vi "SubTRAMAS.vi"(0 "Trama":string) -> (1 "RMC":string[](array[string]), 2 "GGA":string[](array[string]), 3 "GSA":string[](array[string]))   [LabVIEW 2020]
panel:
  out "<CR><LF> GSA":string
  out "<CR><LF> GGA":string
  out "<CR><LF> RMC":string
  out "Estado de navegación RMC":string
  out "Longitud GGA":string
  out "Latitud GGA":string
  out "Longitud RMC":string
  out "Latitud RMC":string
  out "Dilución vertical de precisión GSA":string
  out "Checksum GSA":string
  out "Checksum GGA":string
  out "ID de la estación DGPS GGA":string
  out "Edad DGPS GGA":string
  out "Checksum RMC":string
  out "ID del sistema GNSS GSA":string
  out "Dilución horizontal de precisión GSA":string
  out "Posición dilución de precisión GSA":string
  out "Satelite usado en el canal 12":string
  out "Satelite usado en el canal 11":string
  out "Satelite usado en el canal 10":string
  out "Satelite usado en el canal 9":string
  out "Satelite usado en el canal 8":string
  out "Satelite usado en el canal 7":string
  out "Satelite usado en el canal 6":string
  out "Satelite usado en el canal 5":string
  out "Satelite usado en el canal 4":string
  out "Satelite usado en el canal 3":string
  out "Satelite usado en el canal 2":string
  out "Satelite usado en el canal 1":string
  out "Fix status GSA":string
  out "Modo":string
  out "Separacion geoide GGA":string
  out "Altitud GGA":string
  out "Fix Status GGA":string
  out "Modo de posicionamiento RMC":string
  out "Variacion magnetica RMC":string
  out "Variacion  RMC":string
  out "COG RMC":string
  out "HDOP GGA":string
  out "dds 2":dbl
  out "ma 2":dbl
  out "N° satelites en uso GGA":string
  out "Tiempo GGA":string
  out "dds":dbl
  out "ma":dbl
  out "Valida o Invalida? RMC":string
  out "Velocidad RMC":string
  out "Tiempo RMC":string
  out "Fecha RMC":string
  # "RMC"
  # "GGA"
  # "GSA"
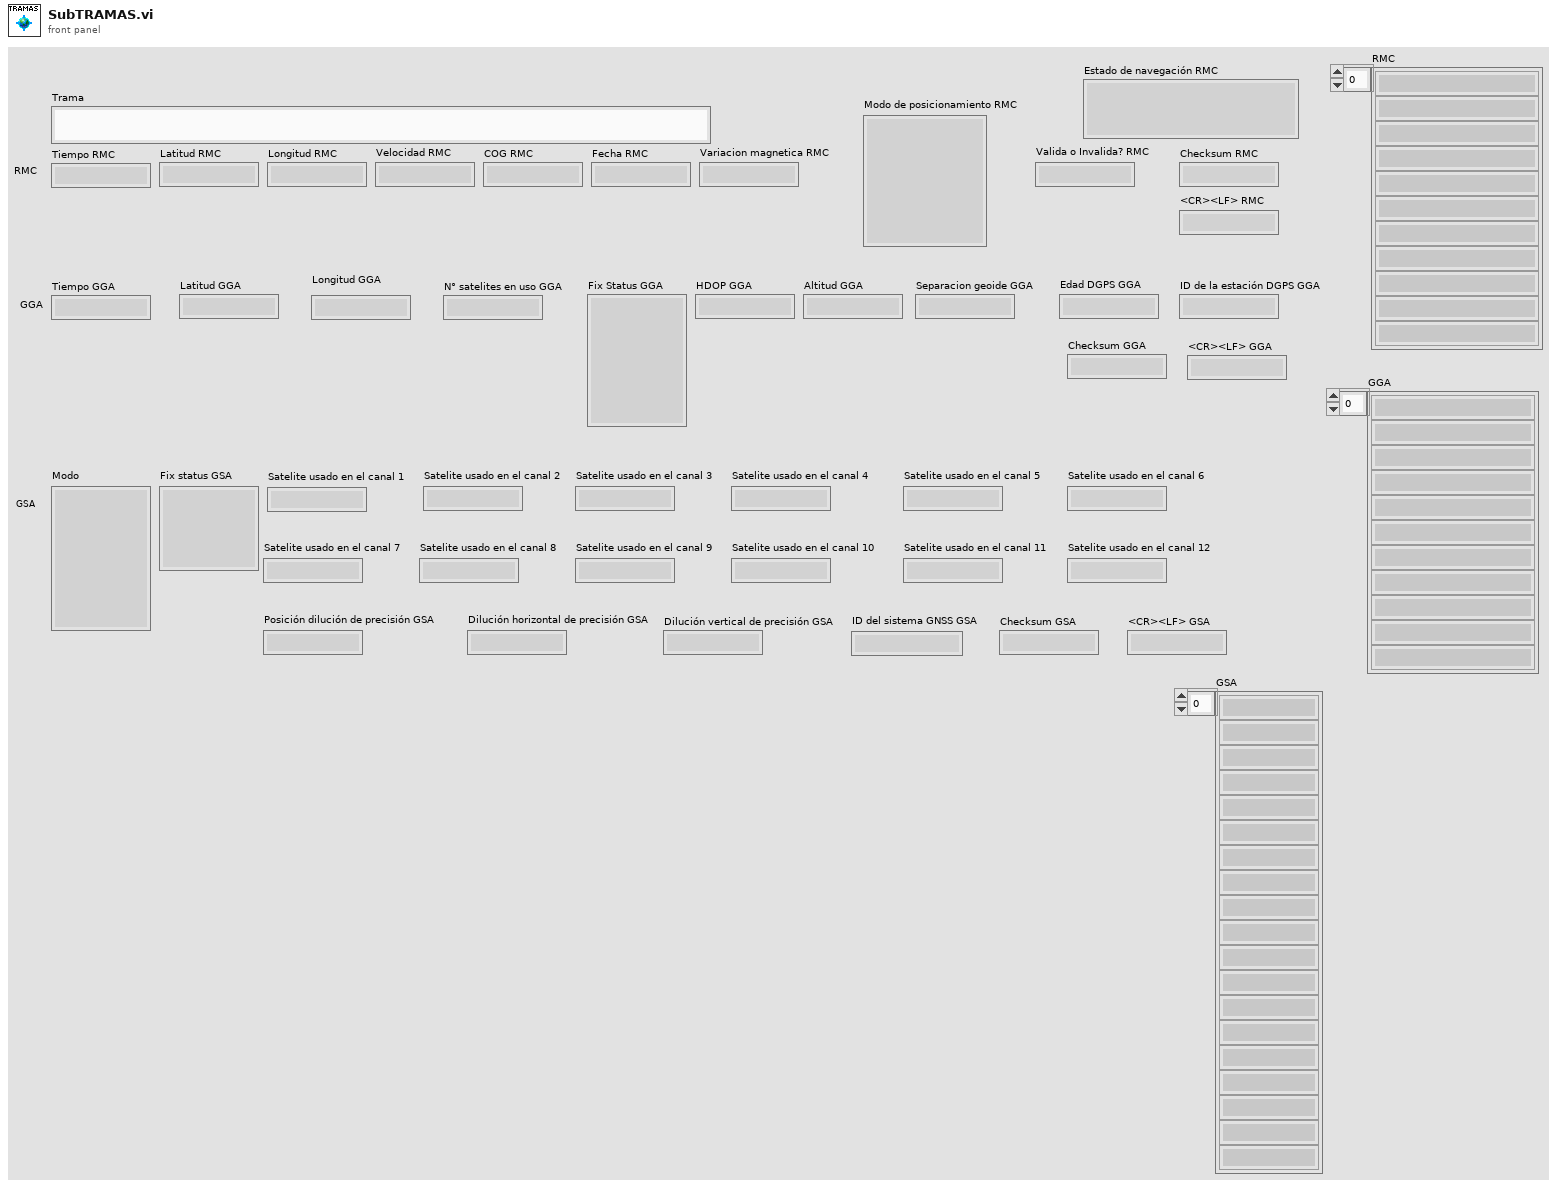
[diagram p1: front panel]
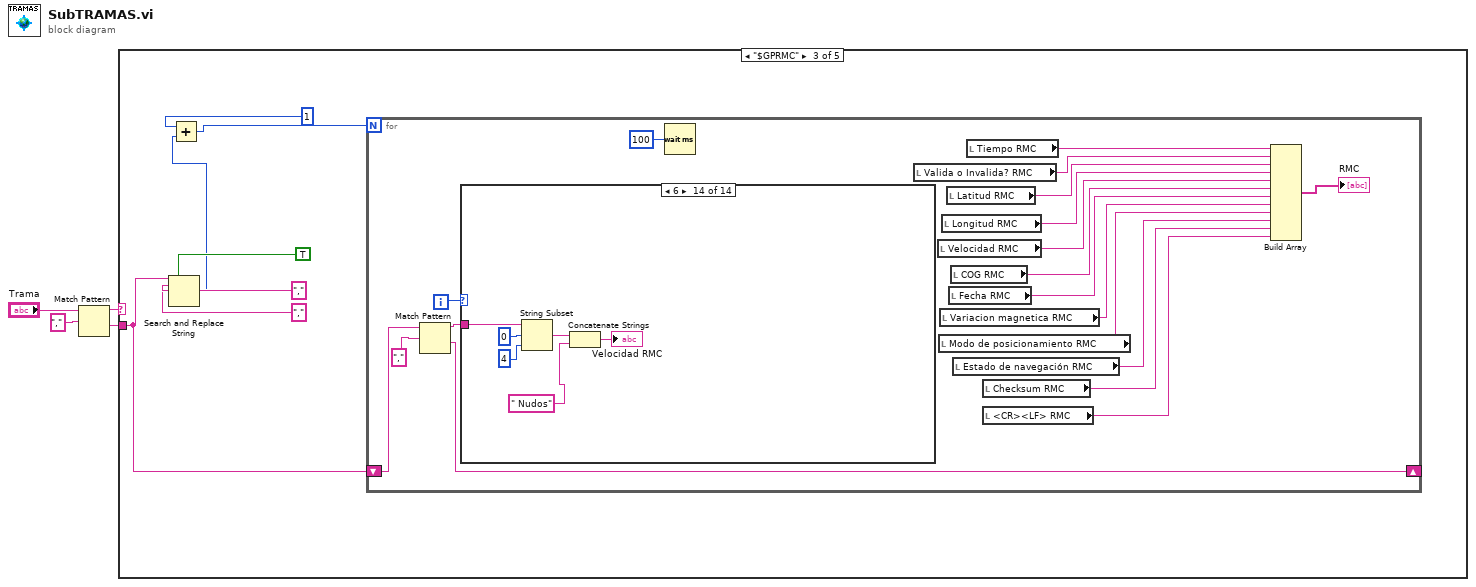
[diagram p0: block diagram]
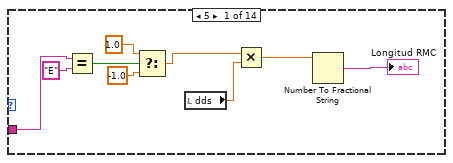
[diagram p4: hidden frame]
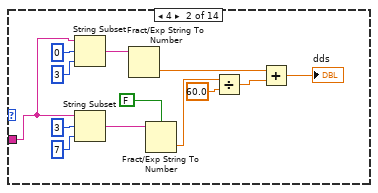
[diagram p5: hidden frame]
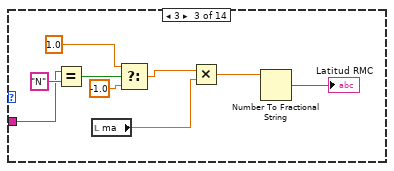
[diagram p6: hidden frame]
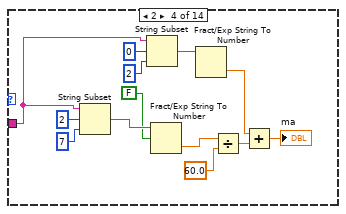
[diagram p7: hidden frame]
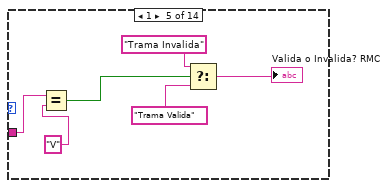
[diagram p8: hidden frame]
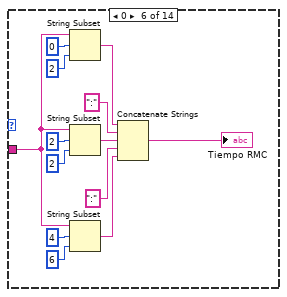
[diagram p9: hidden frame]
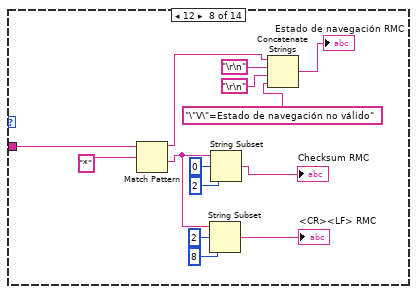
[diagram p11: hidden frame]
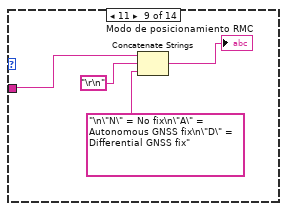
[diagram p12: hidden frame]
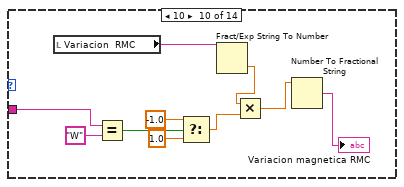
[diagram p13: hidden frame]
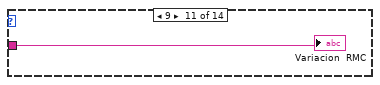
[diagram p14: hidden frame]
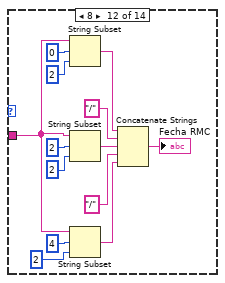
[diagram p15: hidden frame]
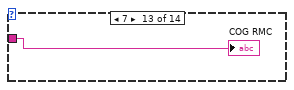
[diagram p16: hidden frame]
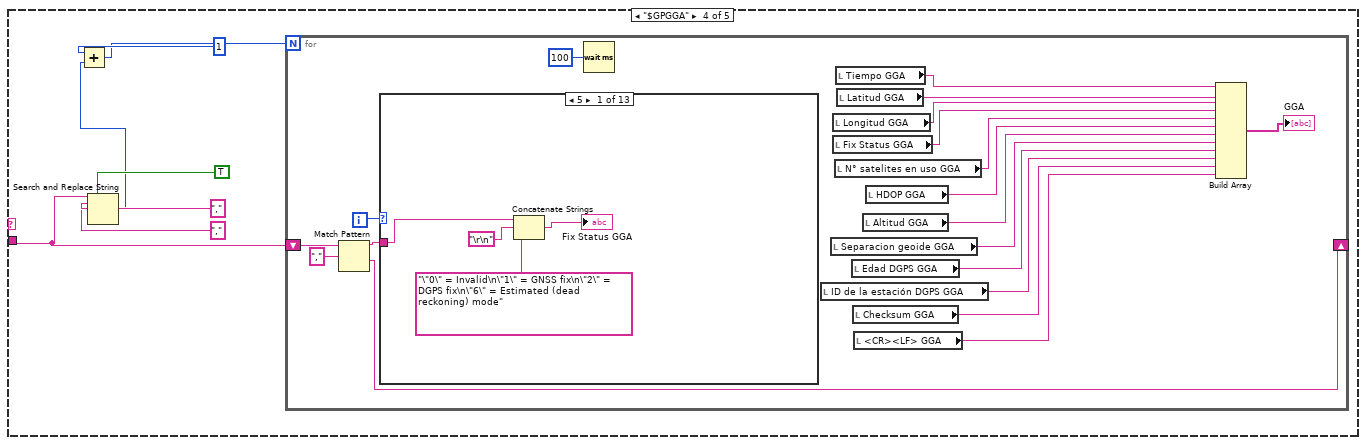
[diagram p17: hidden frame]
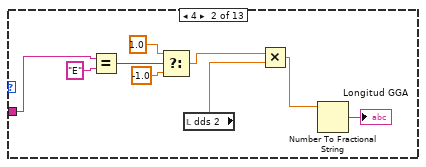
[diagram p18: hidden frame]
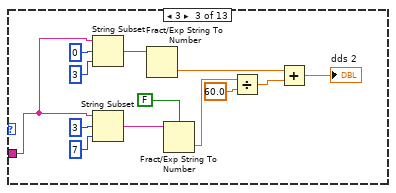
[diagram p19: hidden frame]
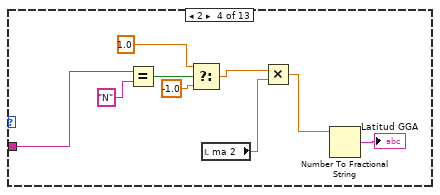
[diagram p20: hidden frame]
diagram:
  n1 = Match Pattern(string="Trama", regular expression=",") -> (before substring=w3:string, after substring=w2:string)  [unwired: 1 in, 2 out]
  n2 = case shown="\"$GPRMC\"" w3 {
    tunnel: w2 -> [_ _ w9 w146 w248]
    frame "False", Default {
    }
    frame "True" {
    }
    frame "$GPRMC" {
      n3 = Search and Replace String(replace all?=TRUE ("replace all? (F)"), input string=w9, search string=",", replace string="," ("replace string (\"\")")) -> (number of replacements=w6:i32)  [unwired: 4 in, 3 out]
      n4 = Add(x=1, y=w6) -> (x+y=w5:i32)
      n5 = for {
        N: w5 -> [_]
        shift-right: [w26] -> _
        shift-left: w9 -> [w29]
        i -> [w28]
        n6 = Match Pattern(string=w29, regular expression=",") -> (before substring=w27:string, after substring=w26:string)  [unwired: 1 in, 2 out]
        n7 = case shown="6" w28 {
          tunnel: w27 -> [w34 w41 w58 w63 w77 w82 _ w106 w110 w116 w122 w124 w136 w138]
          frame 5 {
            n8 = Equal?(x=w34, y="E") -> (x = y?=w37:bool)
            n9 = Select(t=1.0, s=w37, f=-1.0) -> (s? t:f=w35:dbl)
            n10 = local read "dds"() -> (w33:dbl)
            n11 = Multiply(x=w35, y=w33) -> (x*y=w32:dbl)
            n12 = Number To Fractional String(number=w32) -> (F-format string=→"Longitud RMC":string)  [unwired: 3 in]
          }
          frame 4 {
            n13 = String Subset(string=w41, offset (0)=0, length (rest)=3 ("length (rest)")) -> (substring=w52:string)
            n14 = String Subset(string=w41, offset (0)=3, length (rest)=7 ("length (rest)")) -> (substring=w48:string)
            n15 = Fract/Exp String To Number(string=w52) -> (number=w43:dbl)  [unwired: 3 in, 1 out]
            n16 = Fract/Exp String To Number(use system decimal point (T)=FALSE, string=w48) -> (number=w50:dbl)  [unwired: 2 in, 1 out]
            n17 = Divide(x=w50, y=60.0) -> (x/y=w42:dbl)
            n18 = Add(x=w43, y=w42) -> (x+y=→"dds":dbl)
          }
          frame 3 {
            n19 = Equal?(x=w58, y="N") -> (x = y?=w60:bool)
            n20 = local read "ma"() -> (w55:dbl)
            n21 = Select(t=1.0, s=w60, f=-1.0) -> (s? t:f=w56:dbl)
            n22 = Multiply(x=w56, y=w55) -> (x*y=w54:dbl)
            n23 = Number To Fractional String(number=w54) -> (F-format string=→"Latitud RMC":string)  [unwired: 3 in]
          }
          frame 2 {
            n24 = String Subset(string=w63, offset (0)=2, length (rest)=7 ("length (rest)")) -> (substring=w70:string)
            n25 = String Subset(string=w63, offset (0)=0, length (rest)=2 ("length (rest)")) -> (substring=w65:string)
            n26 = Fract/Exp String To Number(use system decimal point (T)=FALSE, string=w70) -> (number=w68:dbl)  [unwired: 2 in, 1 out]
            n27 = Fract/Exp String To Number(string=w65) -> (number=w64:dbl)  [unwired: 3 in, 1 out]
            n28 = Divide(x=w68, y=60.0) -> (x/y=w66:dbl)
            n29 = Add(x=w64, y=w66) -> (x+y=→"ma":dbl)
          }
          frame 1 {
            n30 = Equal?(x=w77, y="V") -> (x = y?=w75:bool)
            n31 = Select(t="Trama Invalida", s=w75, f="Trama Valida") -> (s? t:f=→"Valida o Invalida? RMC":string)
          }
          frame 0 {
            n32 = String Subset(string=w82, offset (0)=0, length (rest)=2 ("length (rest)")) -> (substring=w87:string)
            n33 = String Subset(string=w82, offset (0)=2, length (rest)=2 ("length (rest)")) -> (substring=w85:string)
            n34 = String Subset(string=w82, offset (0)=4, length (rest)=6 ("length (rest)")) -> (substring=w83:string)
            n35 = Concatenate Strings(w87, ":" ("string"), w85, ":" ("string"), w83) -> (→"Tiempo RMC":string)
          }
          frame 20, Default {
          }
          frame 12 {
            n36 = Match Pattern(string=w106, regular expression="*") -> (before substring=w102:string, after substring=w100:string)  [unwired: 1 in, 2 out]
            n37 = String Subset(string=w100, offset (0)=2, length (rest)=8 ("length (rest)")) -> (substring=→"<CR><LF> RMC":string)
            n38 = String Subset(string=w100, offset (0)=0, length (rest)=2 ("length (rest)")) -> (substring=→"Checksum RMC":string)
            n39 = Concatenate Strings(w102, "\r\n", "\r\n", "\"V\"=Estado de navegación no válido") -> (→"Estado de navegación RMC":string)
          }
          frame 11 {
            n40 = Concatenate Strings(w110, "\r\n", "\n\"N\" = No fix\n\"A\" = Autonomous GNSS fix\n\"D\" = Differential GNSS fix") -> (→"Modo de posicionamiento RMC":string)
          }
          frame 10 {
            n41 = local read "Variacion  RMC"() -> (w115:string)
            n42 = Equal?(x=w116, y="W") -> (x = y?=w120:bool)
            n43 = Select(t=-1.0, s=w120, f=1.0) -> (s? t:f=w117:dbl)
            n44 = Fract/Exp String To Number(string=w115) -> (number=w114:dbl)  [unwired: 3 in, 1 out]
            n45 = Multiply(x=w114, y=w117) -> (x*y=w113:dbl)
            n46 = Number To Fractional String(number=w113) -> (F-format string=→"Variacion magnetica RMC":string)  [unwired: 3 in]
          }
          frame 9 {
            "Variacion  RMC" <- w122
          }
          frame 8 {
            n47 = String Subset(string=w124, offset (0)=0, length (rest)=2 ("length (rest)")) -> (substring=w130:string)
            n48 = String Subset(string=w124, offset (0)=2, length (rest)=2 ("length (rest)")) -> (substring=w128:string)
            n49 = String Subset(string=w124, offset (0)=4, length (rest)=2 ("length (rest)")) -> (substring=w126:string)
            n50 = Concatenate Strings(w130, "/" ("string"), w128, "/" ("string"), w126) -> (→"Fecha RMC":string)
          }
          frame 7 {
            "COG RMC" <- w136
          }
          frame 6 {
            n51 = String Subset(string=w138, offset (0)=0, length (rest)=4 ("length (rest)")) -> (substring=w140:string)
            n52 = Concatenate Strings(w140, " Nudos") -> (→"Velocidad RMC":string)
          }
        }
        n53 = Wait (ms)(milliseconds to wait=u32 100) -> ()  [unwired: 1 out]
        n54 = local read "Valida o Invalida? RMC"() -> (w22:string)
        n55 = local read "Velocidad RMC"() -> (w19:string)
        n56 = local read "Modo de posicionamiento RMC"() -> (w15:string)
        n57 = local read "Variacion magnetica RMC"() -> (w16:string)
        n58 = local read "Longitud RMC"() -> (w20:string)
        n59 = local read "Latitud RMC"() -> (w21:string)
        n60 = local read "Fecha RMC"() -> (w17:string)
        n61 = local read "COG RMC"() -> (w18:string)
        n62 = local read "Estado de navegación RMC"() -> (w14:string)
        n63 = local read "Tiempo RMC"() -> (w24:string)
        n64 = local read "Checksum RMC"() -> (w13:string)
        n65 = local read "<CR><LF> RMC"() -> (w12:string)
        n66 = Build Array(w24, w22, w21, w20, w19, w18, w17, w16, w15, w14, w13, w12) -> (→"RMC":string[])
      }
    }
    frame "$GPGGA" {
      n67 = Search and Replace String(replace all?=TRUE ("replace all? (F)"), input string=w146, search string=",", replace string="," ("replace string (\"\")")) -> (number of replacements=w144:i32)  [unwired: 4 in, 3 out]
      n68 = Add(x=1, y=w144) -> (x+y=w143:i32)
      n69 = for {
        N: w143 -> [_]
        shift-right: [w164] -> _
        shift-left: w146 -> [w167]
        i -> [w166]
        n70 = Match Pattern(string=w167, regular expression=",") -> (before substring=w165:string, after substring=w164:string)  [unwired: 1 in, 2 out]
        n71 = case shown="5" w166 {
          tunnel: w165 -> [w172 w176 w182 w198 w209 w217 _ w238 w240 w241 w242 w243 w244]
          frame 5 {
            n72 = Concatenate Strings(w172, "\r\n", "\"0\" = Invalid\n\"1\" = GNSS fix\n\"2\" = DGPS fix\n\"6\" = Estimated (dead reckoning) mode") -> (→"Fix Status GGA":string)
          }
          frame 4 {
            n73 = Equal?(x=w176, y="E") -> (x = y?=w179:bool)
            n74 = Select(t=1.0, s=w179, f=-1.0) -> (s? t:f=w177:dbl)
            n75 = local read "dds 2"() -> (w175:dbl)
            n76 = Multiply(x=w177, y=w175) -> (x*y=w174:dbl)
            n77 = Number To Fractional String(number=w174) -> (F-format string=→"Longitud GGA":string)  [unwired: 3 in]
          }
          frame 3 {
            n78 = String Subset(string=w182, offset (0)=0, length (rest)=3 ("length (rest)")) -> (substring=w194:string)
            n79 = String Subset(string=w182, offset (0)=3, length (rest)=7 ("length (rest)")) -> (substring=w190:string)
            n80 = Fract/Exp String To Number(string=w194) -> (number=w185:dbl)  [unwired: 3 in, 1 out]
            n81 = Fract/Exp String To Number(use system decimal point (T)=FALSE, string=w190) -> (number=w192:dbl)  [unwired: 2 in, 1 out]
            n82 = Divide(x=w192, y=60.0) -> (x/y=w184:dbl)
            n83 = Add(x=w185, y=w184) -> (x+y=→"dds 2":dbl)
          }
          frame 2 {
            n84 = Equal?(x=w198, y="N") -> (x = y?=w202:bool)
            n85 = Select(t=1.0, s=w202, f=-1.0) -> (s? t:f=w199:dbl)
            n86 = local read "ma 2"() -> (w197:dbl)
            n87 = Multiply(x=w199, y=w197) -> (x*y=w196:dbl)
            n88 = Number To Fractional String(number=w196) -> (F-format string=→"Latitud GGA":string)  [unwired: 3 in]
          }
          frame 1 {
            n89 = String Subset(string=w209, offset (0)=2, length (rest)=7 ("length (rest)")) -> (substring=w214:string)
            n90 = String Subset(string=w209, offset (0)=0, length (rest)=2 ("length (rest)")) -> (substring=w211:string)
            n91 = Fract/Exp String To Number(use system decimal point (T)=FALSE, string=w214) -> (number=w213:dbl)  [unwired: 2 in, 1 out]
            n92 = Fract/Exp String To Number(string=w211) -> (number=w208:dbl)  [unwired: 3 in, 1 out]
            n93 = Divide(x=w213, y=60.0) -> (x/y=w212:dbl)
            n94 = Add(x=w208, y=w212) -> (x+y=→"ma 2":dbl)
          }
          frame 0 {
            n95 = String Subset(string=w217, offset (0)=0, length (rest)=2 ("length (rest)")) -> (substring=w223:string)
            n96 = String Subset(string=w217, offset (0)=2, length (rest)=2 ("length (rest)")) -> (substring=w221:string)
            n97 = String Subset(string=w217, offset (0)=4, length (rest)=6 ("length (rest)")) -> (substring=w219:string)
            n98 = Concatenate Strings(w223, ":" ("string"), w221, ":" ("string"), w219) -> (→"Tiempo GGA":string)
          }
          frame 15, Default {
          }
          frame 13 {
            n99 = Match Pattern(string=w238, regular expression="*") -> (before substring=→"ID de la estación DGPS GGA":string, after substring=w230:string)  [unwired: 1 in, 2 out]
            n100 = String Subset(string=w230, offset (0)=2, length (rest)=8 ("length (rest)")) -> (substring=→"<CR><LF> GGA":string)
            n101 = String Subset(string=w230, offset (0)=0, length (rest)=2 ("length (rest)")) -> (substring=→"Checksum GGA":string)
          }
          frame 12 {
            "Edad DGPS GGA" <- w240
          }
          frame 10 {
            "Separacion geoide GGA" <- w241
          }
          frame 8 {
            "Altitud GGA" <- w242
          }
          frame 7 {
            "HDOP GGA" <- w243
          }
          frame 6 {
            "N° satelites en uso GGA" <- w244
          }
        }
        n102 = Wait (ms)(milliseconds to wait=u32 100) -> ()  [unwired: 1 out]
        n103 = local read "ID de la estación DGPS GGA"() -> (w152:string)
        n104 = local read "Separacion geoide GGA"() -> (w154:string)
        n105 = local read "Longitud GGA"() -> (w159:string)
        n106 = local read "Fix Status GGA"() -> (w158:string)
        n107 = local read "N° satelites en uso GGA"() -> (w157:string)
        n108 = local read "Tiempo GGA"() -> (w162:string)
        n109 = local read "Latitud GGA"() -> (w161:string)
        n110 = local read "Edad DGPS GGA"() -> (w153:string)
        n111 = local read "Checksum GGA"() -> (w151:string)
        n112 = local read "<CR><LF> GGA"() -> (w150:string)
        n113 = local read "Altitud GGA"() -> (w155:string)
        n114 = local read "HDOP GGA"() -> (w156:string)
        n115 = Build Array(w162, w161, w159, w158, w157, w156, w155, w154, w153, w152, w151, w150) -> (→"GGA":string[])
      }
    }
    frame "$GPGSA" {
      n116 = Search and Replace String(replace all?=TRUE ("replace all? (F)"), input string=w248, search string=",", replace string="," ("replace string (\"\")")) -> (number of replacements=w246:i32)  [unwired: 4 in, 3 out]
      n117 = Add(x=1, y=w246) -> (x+y=w247:i32)
      n118 = for {
        N: w247 -> [_]
        shift-right: [w275] -> _
        shift-left: w248 -> [w277]
        i -> [w273]
        n119 = Match Pattern(string=w277, regular expression=",") -> (before substring=w276:string, after substring=w275:string)  [unwired: 1 in, 2 out]
        n120 = case shown="17" w273 {
          tunnel: w276 -> [w279 w280 w281 w282 w286 w292 _ w301 w303 w304 w305 w306 w307 w308 w309 w310 w311 w312 w313]
          frame 5 {
            "Satelite usado en el canal 4" <- w279
          }
          frame 4 {
            "Satelite usado en el canal 3" <- w280
          }
          frame 3 {
            "Satelite usado en el canal 2" <- w281
          }
          frame 2 {
            "Satelite usado en el canal 1" <- w282
          }
          frame 1 {
            n121 = Concatenate Strings(w286, "\r\n", "\r\n", "\"1\" = No fix\n\"2\" = 2D fix\n\"3\" = 3D fix") -> (→"Fix status GSA":string)
          }
          frame 0 {
            n122 = Concatenate Strings(w292, "\r\n", "\r\n", "\"M\"=Manual, forced to switch 2D/3D mode\n\"A\"=Allowed to automatically switch 2D/3D mode") -> (→"Modo":string)
          }
          frame 20, Default {
          }
          frame 17 {
            n123 = Match Pattern(string=w301, regular expression="*") -> (before substring=→"ID del sistema GNSS GSA":string, after substring=w295:string)  [unwired: 1 in, 2 out]
            n124 = String Subset(string=w295, offset (0)=2, length (rest)=8 ("length (rest)")) -> (substring=→"<CR><LF> GSA":string)
            n125 = String Subset(string=w295, offset (0)=0, length (rest)=2 ("length (rest)")) -> (substring=→"Checksum GSA":string)
          }
          frame 16 {
            "Dilución vertical de precisión GSA" <- w303
          }
          frame 15 {
            "Dilución horizontal de precisión GSA" <- w304
          }
          frame 14 {
            "Posición dilución de precisión GSA" <- w305
          }
          frame 13 {
            "Satelite usado en el canal 12" <- w306
          }
          frame 12 {
            "Satelite usado en el canal 11" <- w307
          }
          frame 11 {
            "Satelite usado en el canal 10" <- w308
          }
          frame 10 {
            "Satelite usado en el canal 9" <- w309
          }
          frame 9 {
            "Satelite usado en el canal 8" <- w310
          }
          frame 8 {
            "Satelite usado en el canal 7" <- w311
          }
          frame 7 {
            "Satelite usado en el canal 6" <- w312
          }
          frame 6 {
            "Satelite usado en el canal 5" <- w313
          }
        }
        n126 = Wait (ms)(milliseconds to wait=u32 100) -> ()  [unwired: 1 out]
        n127 = local read "Dilución horizontal de precisión GSA"() -> (w256:string)
        n128 = local read "Dilución vertical de precisión GSA"() -> (w255:string)
        n129 = local read "Posición dilución de precisión GSA"() -> (w257:string)
        n130 = local read "Satelite usado en el canal 1"() -> (w269:string)
        n131 = local read "Satelite usado en el canal 10"() -> (w260:string)
        n132 = local read "Satelite usado en el canal 11"() -> (w259:string)
        n133 = local read "Satelite usado en el canal 12"() -> (w258:string)
        n134 = local read "Satelite usado en el canal 7"() -> (w263:string)
        n135 = local read "Satelite usado en el canal 2"() -> (w268:string)
        n136 = local read "Satelite usado en el canal 3"() -> (w267:string)
        n137 = local read "Satelite usado en el canal 4"() -> (w266:string)
        n138 = local read "Satelite usado en el canal 5"() -> (w265:string)
        n139 = local read "Satelite usado en el canal 6"() -> (w264:string)
        n140 = local read "Satelite usado en el canal 9"() -> (w261:string)
        n141 = local read "Satelite usado en el canal 8"() -> (w262:string)
        n142 = local read "ID del sistema GNSS GSA"() -> (w254:string)
        n143 = local read "Checksum GSA"() -> (w253:string)
        n144 = local read "<CR><LF> GSA"() -> (w252:string)
        n145 = local read "Fix status GSA"() -> (w270:string)
        n146 = local read "Modo"() -> (w272:string)
        n147 = Build Array(w272, w270, w269, w268, w267, w266, w265, w264, w263, w262, w261, w260, w259, w258, w257, w256, w255, w254, w253, w252) -> (→"GSA":string[])
      }
    }
  }
